vi "Dialog_TestGC (SubVI).vi"() -> ()   [LabVIEW 2017]
uses:
  Global_SNK3_HF.vi
  LV_Unicorn/LV_Unicorn.lvlib
panel:
  in  "Атт":u16(ring) items=["0 дБ"=114, "10 дБ"=104, "20 дБ"=94, "30 дБ"=84, "40 дБ"=74, "50 дБ"=64, "60 дБ"=54, "70 дБ"=44, "80 дБ"=34, "90 дБ"=24, "100 дБ"=14, "110 дБ"=4]
  in  "K":dbl
  in  "K_start":dbl min=0.0 max=80.0
  out "Process":bool
  in  "K_finish":dbl=41.0 format="%#_13g"
  in  "Pause":u32=1000 caption="Пауза, мс"
  out "Meas":bool
  out "subarray 3":sgl[](array[numeric])
  out "subarray 2":sgl[](array[numeric])
  in  "ResetCalCoeff":bool
  in  "index":i32=1 min=1 max=2 step=1
  out "subarray":sgl[](array[numeric])
  in  "WriteCalCoeff":bool
  in  "ReadCalCoeff":bool
  in  "StopMeas":bool
  in  "StartMeas":bool
  in  "Exit":bool
  in  "Coeff":bool
  in  "Tab Control":enum32{"Page 1", "Page 2", "Page 3"}(tab)
  out "TimeMeasStart":u32
  out "Gain0":dbl caption="Усиление 1, дБ" min=0.0 max=80.0 step=1.0 format="%.1g"
  out "Gain1":dbl caption="Усиление 2, дБ" min=0.0 max=80.0 step=1.0 format="%.1g"
  in  "Tick":i32=1 caption="№ такта" min=1 max=32 step=1
  out "TableMeasAmpl":string[][](table)=[["0.000000E+0", "2.352698E-3", "2.352698E-3"], ["1.000000E+0", "2.227753E-3", "2.227753E-3"], ["2.000000E+0", "2.159166E-3", "2.159166E-3"], ["3.000000E+0", "2.145925E-3", "2.145925E-3"], ["4.000000E+0", "2.185622E-3", "2.185622E-3"], ["5.000000E+0", "2.219339E-3", "2.219339E-3"], ["6.000000E+0", "2.237044E-3", "2.237044E-3"], ["7.000000E+0", "2.206156E-3", "2.206156E-3"], ["8.000000E+0", "2.176003E-3", "2.176003E-3"], ["9.000000E+0", "2.179087E-3", "2.179087E-3"], ["1.000000E+1", "2.224777E-3", "2.224777E-3"], ["1.100000E+1", "2.236265E-3", "2.236265E-3"], ["1.200000E+1", "2.240637E-3", "2.240637E-3"], ["1.300000E+1", "2.236521E-3", "2.236521E-3"], ["1.400000E+1", "2.209496E-3", "2.209496E-3"], ["1.500000E+1", "2.200976E-3", "2.200976E-3"], ["1.600000E+1", "2.243053E-3", "2.243053E-3"], ["1.700000E+1", "2.254625E-3", "2.254625E-3"], ["1.800000E+1", "2.279993E-3", "2.279993E-3"], ["1.900000E+1", "2.248004E-3", "2.248004E-3"], ["2.000000E+1", "2.239042E-3", "2.239042E-3"], ["2.100000E+1", "2.234369E-3", "2.234369E-3"], ["2.200000E+1", "2.262064E-3", "2.262064E-3"], ["2.300000E+1", "2.298454E-3", "2.298454E-3"], ["2.400000E+1", "2.297119E-3", "2.297119E-3"], ["2.500000E+1", "2.286266E-3", "2.286266E-3"], ["2.600000E+1", "2.257747E-3", "2.257747E-3"], ["2.700000E+1", "2.267244E-3", "2.267244E-3"], ["2.800000E+1", "2.308694E-3", "2.308694E-3"], ["2.900000E+1", "2.314665E-3", "2.314665E-3"], ["3.000000E+1", "2.329444E-3", "2.329444E-3"], ["3.100000E+1", "2.315041E-3", "2.315041E-3"], ["3.200000E+1", "2.303474E-3", "2.303474E-3"], ["3.300000E+1", "2.340175E-3", "2.340175E-3"], ["3.400000E+1", "2.384913E-3", "2.384913E-3"], ["3.500000E+1", "2.422117E-3", "2.422117E-3"], ["3.600000E+1", "2.405179E-3", "2.405179E-3"], ["3.700000E+1", "2.373606E-3", "2.373606E-3"], ["3.800000E+1", "2.375906E-3", "2.375906E-3"], ["3.900000E+1", "2.410228E-3", "2.410228E-3"], ["4.000000E+1", "2.466864E-3", "2.466864E-3"]]
  in  "GainSlopePL0":sgl=48.8 format="%_4g"
  in  "GainSlopePL1":sgl=48.8 format="%_4g"
  in  "GainOffsetPL0":sgl=1.12 format="%_4g"
  in  "GainOffsetPL1":sgl=1.12 format="%_4g"
  out "Time":u32
  out "Bode":cluster{dbl[], dbl[]}[](graph) caption="XY Graph - Dark"
  out "Array":sgl[][](array[numeric])
  out "GainCorrectionMeas":dbl[][](array[numeric])=[[0.0, 1.0, 2.0, 3.0, 4.0, 5.0, 6.0, 7.0, 8.0, 9.0, 10.0, 11.0, 12.0, 13.0, 14.0, 15.0, 16.0, 17.0, 18.0, 19.0, 20.0, 21.0, 22.0, 23.0, 24.0, 25.0, 26.0, 27.0, 28.0, 29.0, 30.0, 31.0, 32.0, 33.0, 34.0, 35.0, 36.0, 37.0, 38.0, 39.0, 40.0], [-11.232429740269282, -12.70452761402231, -11.319398282381112, -8.995224772277945, -8.870021411520888, -9.034168301334523, -6.792608737521233, -6.370422166599608, -5.823648015304537, -3.66807443072101, -3.031280637510223, -2.0516253300602667, -2.1317894897174536, 0.4940671061840171, 0.61634452640758, 1.0717510423645895, 4.213932160484772, 4.150072217304057, 4.823706052399056, 6.634471019075436, 7.0919550396868996, 8.35048456573561, 10.394659114064568, 10.34651220779031, 10.155847449848958, 11.22080285980282, 12.73098000476622, 13.476154286586526, 13.37702273588783, 15.066209323545356, 16.361307543145575, 17.17482761716563, 17.245659942964423, 18.27256109717559, 18.698807995907593, 18.073313398218705, 18.77836596615101, 19.022884569212057, 18.781051489757388, 19.253641064117456, 20.313889900641513], [-0.02984003478187235, 0.024395588662363472, -0.026881785088726566, -0.01479701311601106, 0.0070473626365402334, -0.04659877911303749, -0.016585774038287197, -0.035195931797667335, 0.018367098970756415, -0.011084536358572277, 0.01184492173421488, 0.008921059976523088, -0.0014462769298614377, -0.010460598191466323, 0.007060342982912368, 0.007319953984052665, 0.0004817943251253796, -0.008217073037779824, 0.010773518388668994, -0.02068839120505336, -0.021134773648135673, 0.007815399845050284, -0.0006033387891328663, -0.009914345630571161, -0.001809363536513138, 0.01397513427572345, 0.011453140739196645, 0.007103610944255908, 0.00231083143198487, -0.0019520005509407457, 0.008239472023896544, 0.011243188031017266, 0.017396690794598844, -0.004540671429712696, 0.003022227667659586, 0.0065086953679980054, 0.05257819699592949, -0.004117202098556384, 0.012485662438209155, 0.02089110110227745, -0.004640054097832816]]
  out "Array 2":sgl[][](array[numeric])
  in  "ClearTableMeasAmpl":bool
  in  "ViewGraf":bool
  in  "ToExcelTable":bool
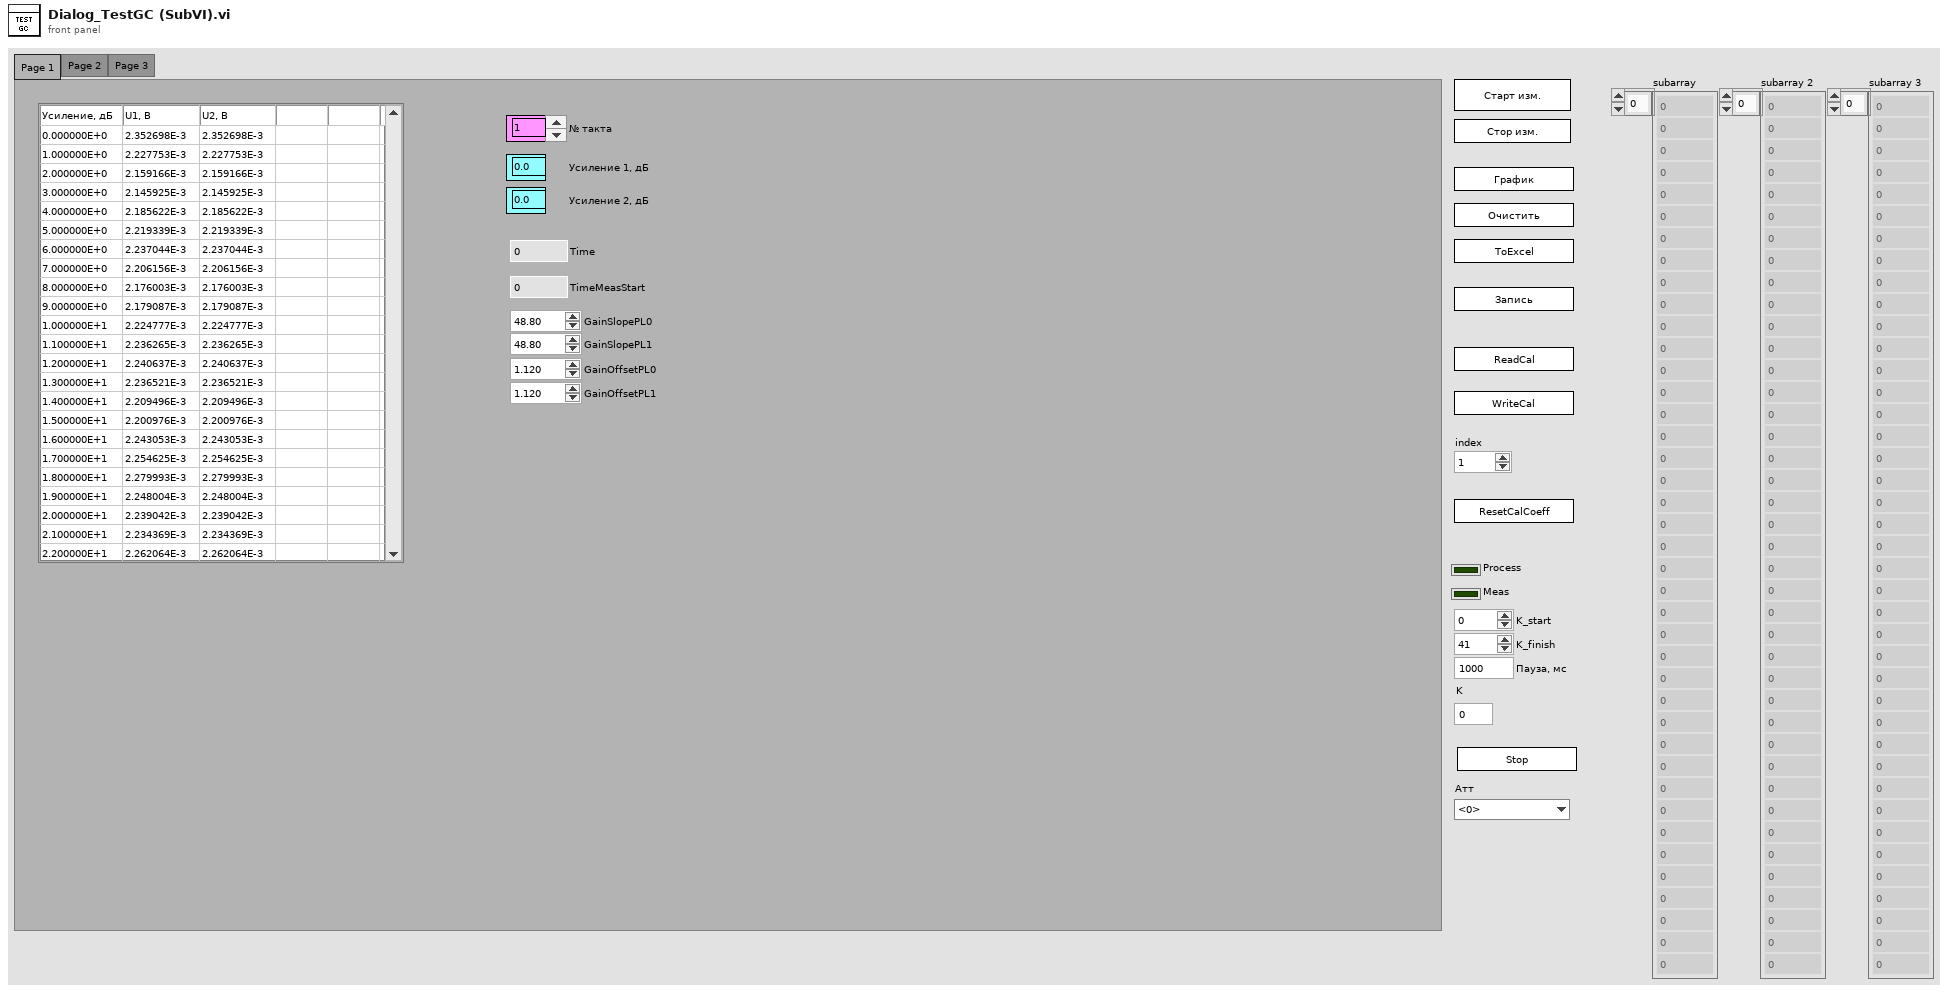
[diagram p1: front panel]
types:
  T1 = typedef "MeasControl.ctl" = cluster{"FFT amplitude":dbl, "amplitude":dbl, "RMS":dbl, "detected frequency":dbl, "way sensor 1":ext, "way sensor 2":ext, "detected frequency 2":dbl, "time trig":dbl, "time trig 2":dbl, "DC":dbl, "trigger detected?":bool, "FFT amplitude mean":dbl}
  T2 = typedef "LV_Unicorn.lvlib/unicorn_Param.ctl" = cluster{"conParam":T3, "Param":T4}
  T3 = typedef "LV_Unicorn.lvlib/unicorn_conn.ctl" = cluster{"ReadIntParam":bool, "ReadDescrParam":bool, "ReadFloatParam":bool, "debug":bool, "ReadJSON":bool, "IP_address":string, "N_attempts":i32, "type_con":enum16{"Serial", "TCP"}, "MB_address":i32, "VISA":refnum<visa-resource-name>, "connection ID":refnum<k5>, "nameDevices":string, "timeout":i32, "port":u16, "type_version":string, "baud_rate":u32, "VersionControl":bool, "TCP_conn":bool, "WindowSize":i32}
  T4 = typedef "LV_Unicorn.lvlib/unicorn_JSON.ctl" = cluster{"NumParam":cluster{"NTelem":i32, "NInt":i32, "NFloat":i32, "NTable":i32}, "ParamInt":T5, "Telemetry":T6, "Table":T7, "ParamFloat":T8}
  T5 = typedef "LV_Unicorn.lvlib/unicorn_ParamInt.ctl" = cluster{"ID":string, "Num":i32, "Name":string, "Type":string, "Enum":string, "Desc":string, "Unit":string, "Access":string, "FormatStr":string, "Min":i32, "Max":i32}[]
  T6 = typedef "LV_Unicorn.lvlib/unicorn_Telemetry.ctl" = cluster{"ID":string, "Num":i32, "Name":string, "Desc":string, "Unit":string, "FormatStr":string, "Min":i32, "Max":i32}[]
  T7 = typedef "LV_Unicorn.lvlib/unicorn_Table.ctl" = cluster{"Num":i32, "Access":string, "ColumnCount":i32, "NeedParamPrepare":bool, "Columns":cluster{"Column":i32, "Desc":string, "Name":string}[], "DataType":string, "FormatStr":string, "ID":string, "Name":string, "RowCount":i32, "Rows":cluster{"Desc":string, "ID":string, "Max":i32, "Min":i32, "Name":string, "Row":i32, "Unit":string}[], "Type":string}[]
  T8 = typedef "LV_Unicorn.lvlib/unicorn_ParamFloat.ctl" = cluster{"ID":string, "Num":i32, "Name":string, "Type":string, "Enum":string, "Desc":string, "Unit":string, "Access":string, "FormatStr":string, "Min":sgl, "Max":sgl}[]
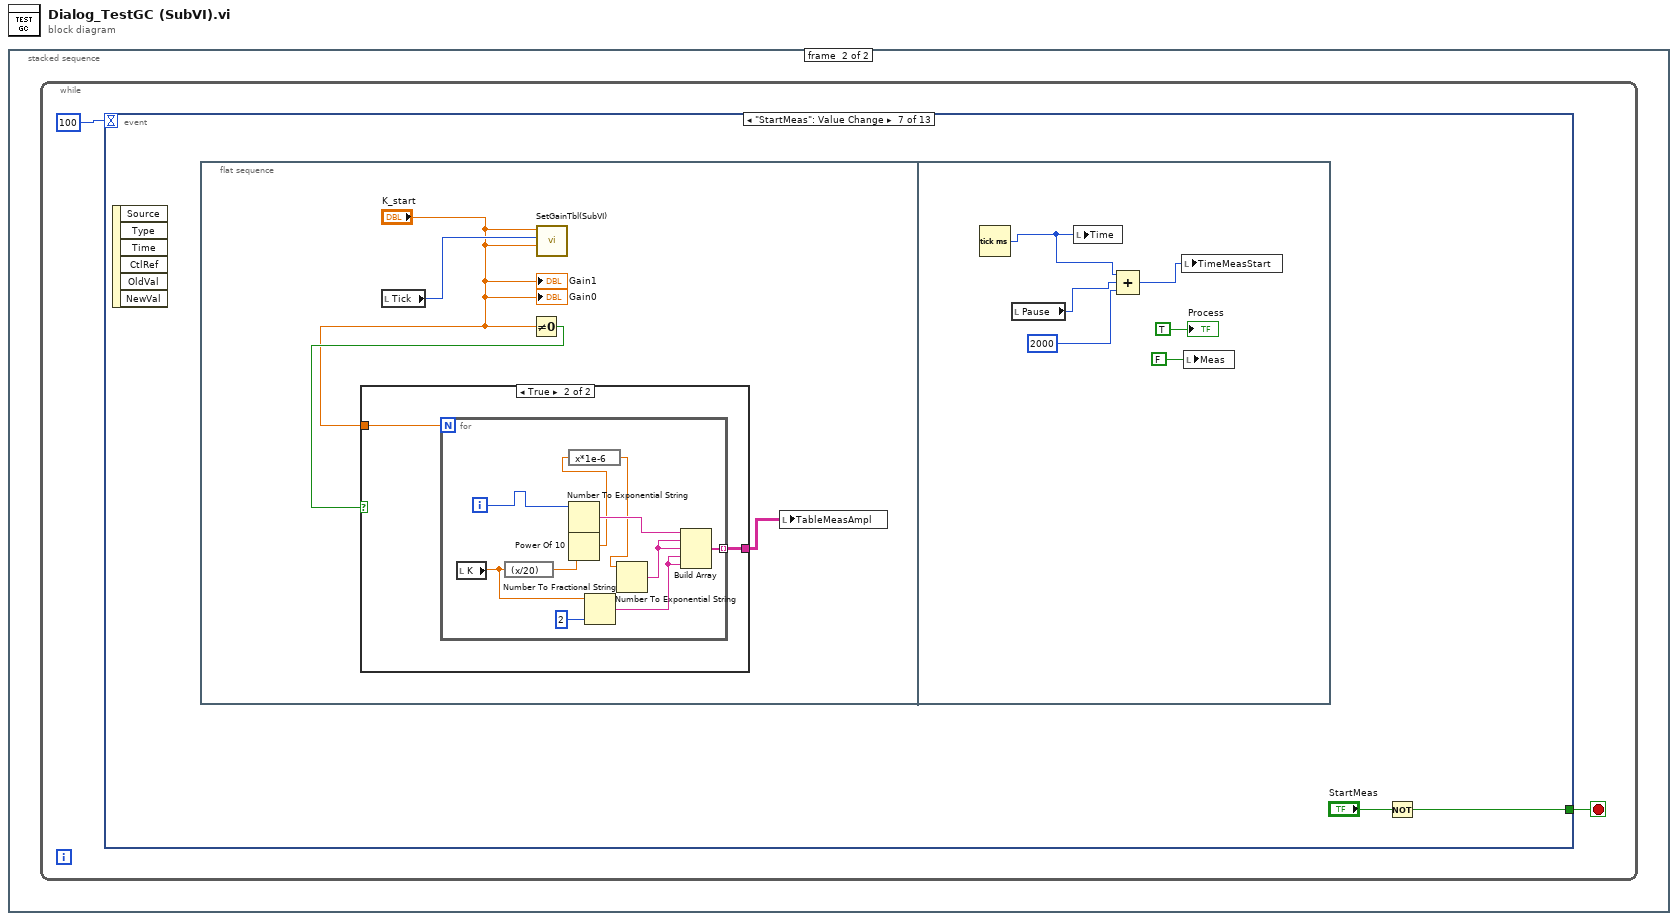
[diagram p0: block diagram]
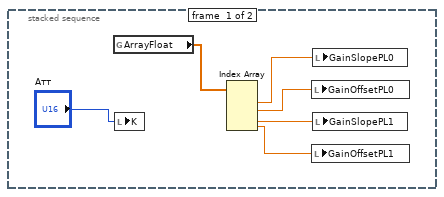
[diagram p2: hidden frame]
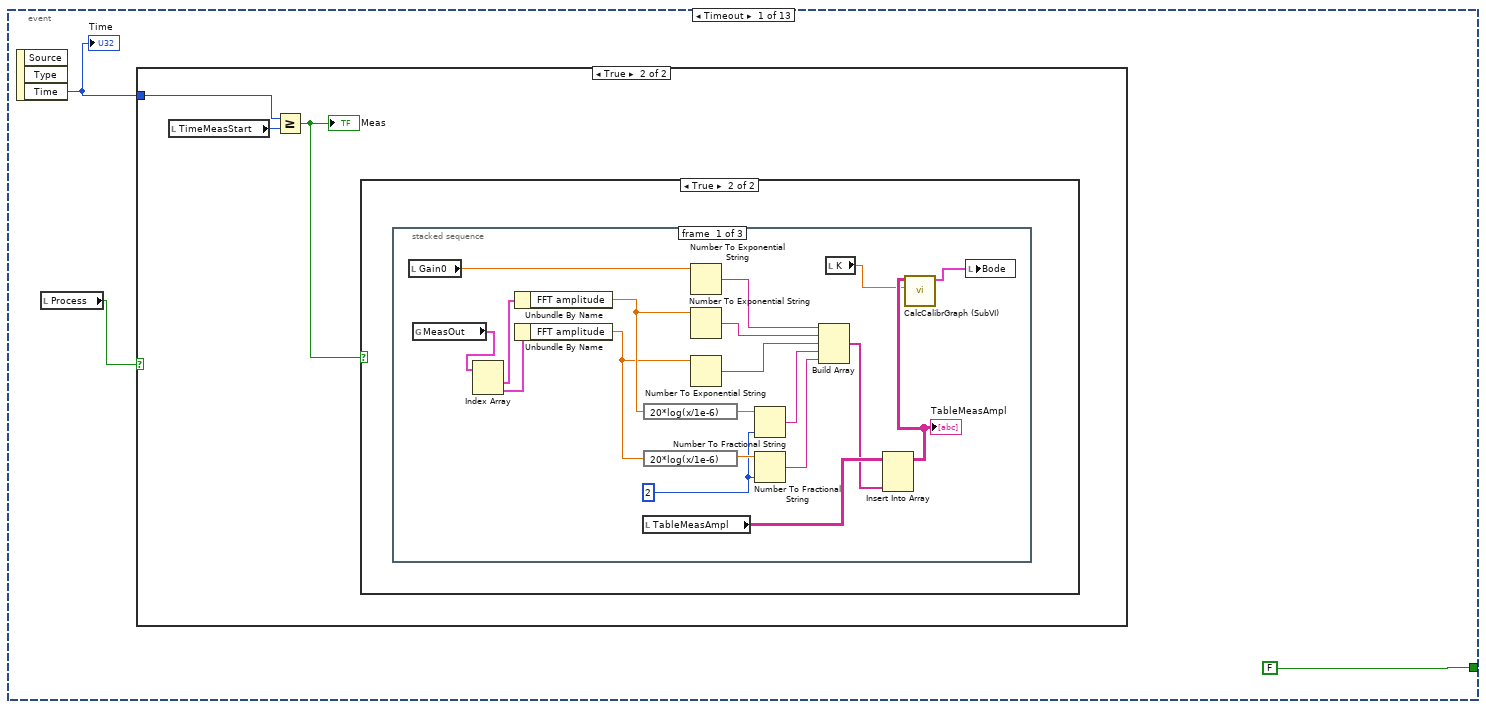
[diagram p3: hidden frame]
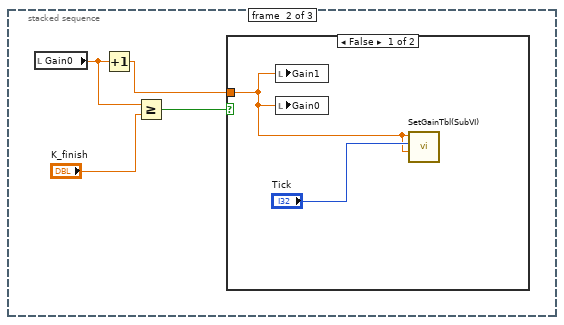
[diagram p6: hidden frame]
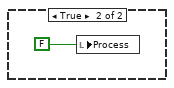
[diagram p7: hidden frame]
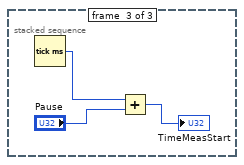
[diagram p8: hidden frame]
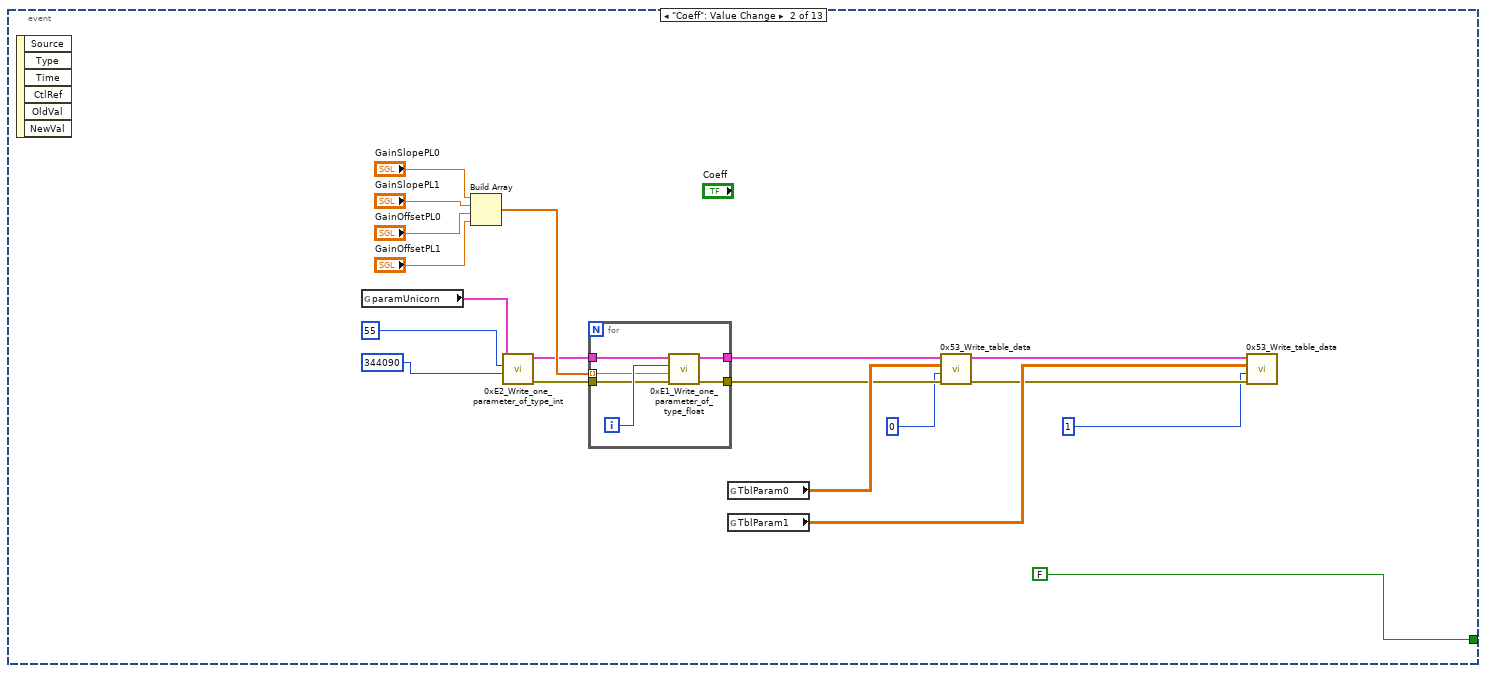
[diagram p9: hidden frame]
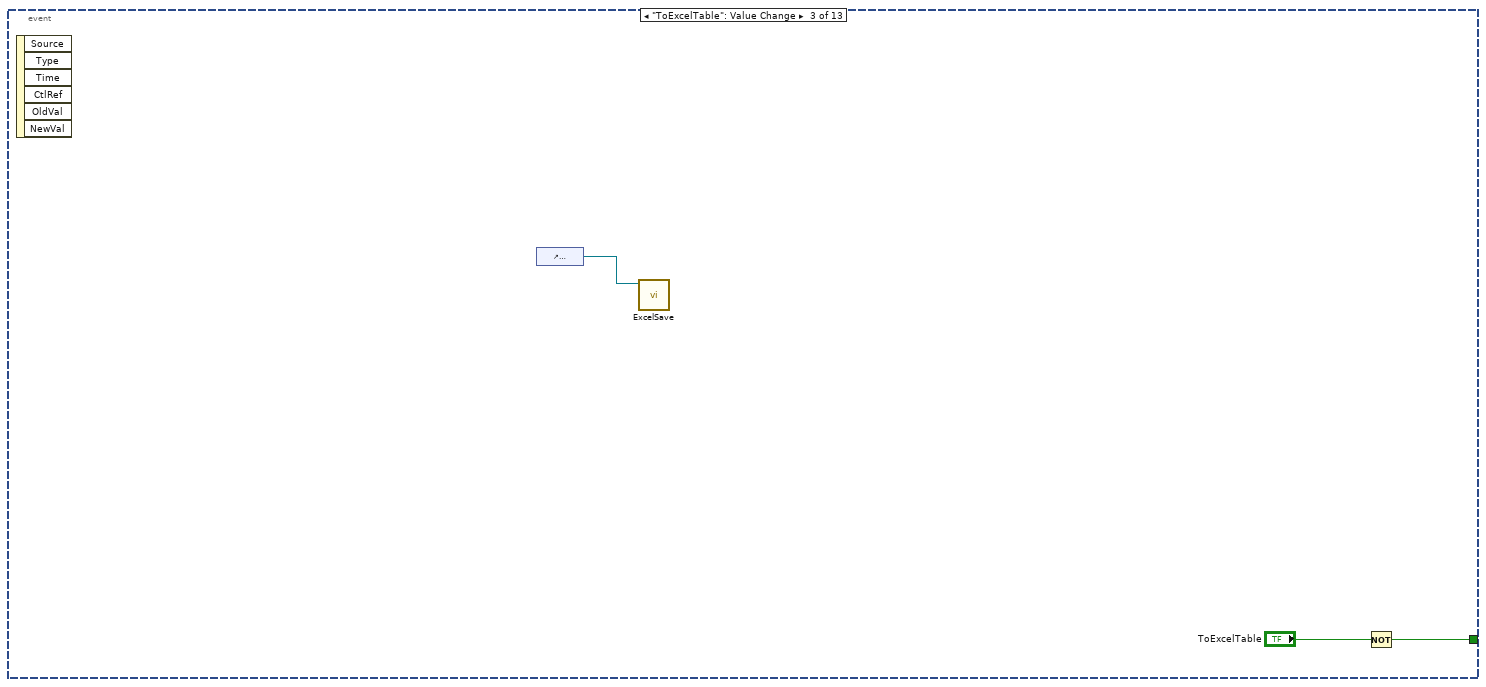
[diagram p10: hidden frame]
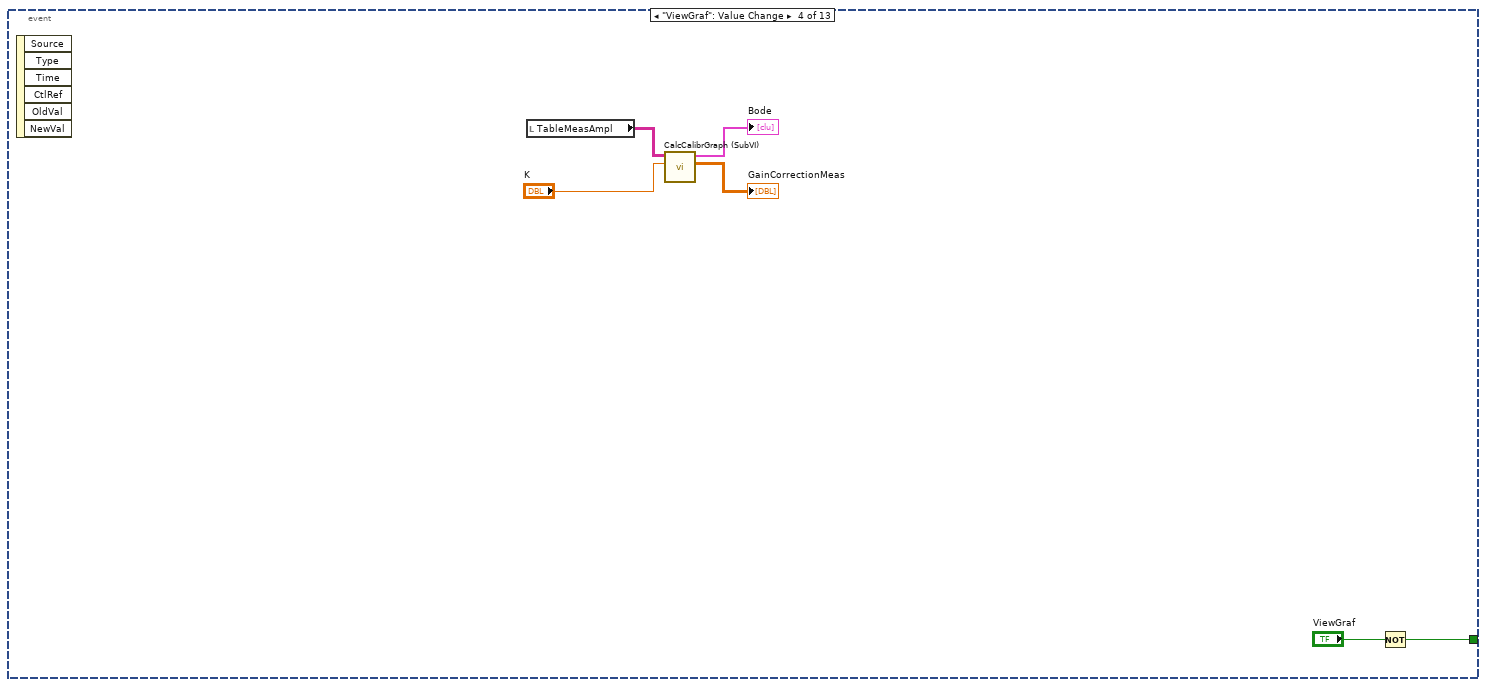
[diagram p11: hidden frame]
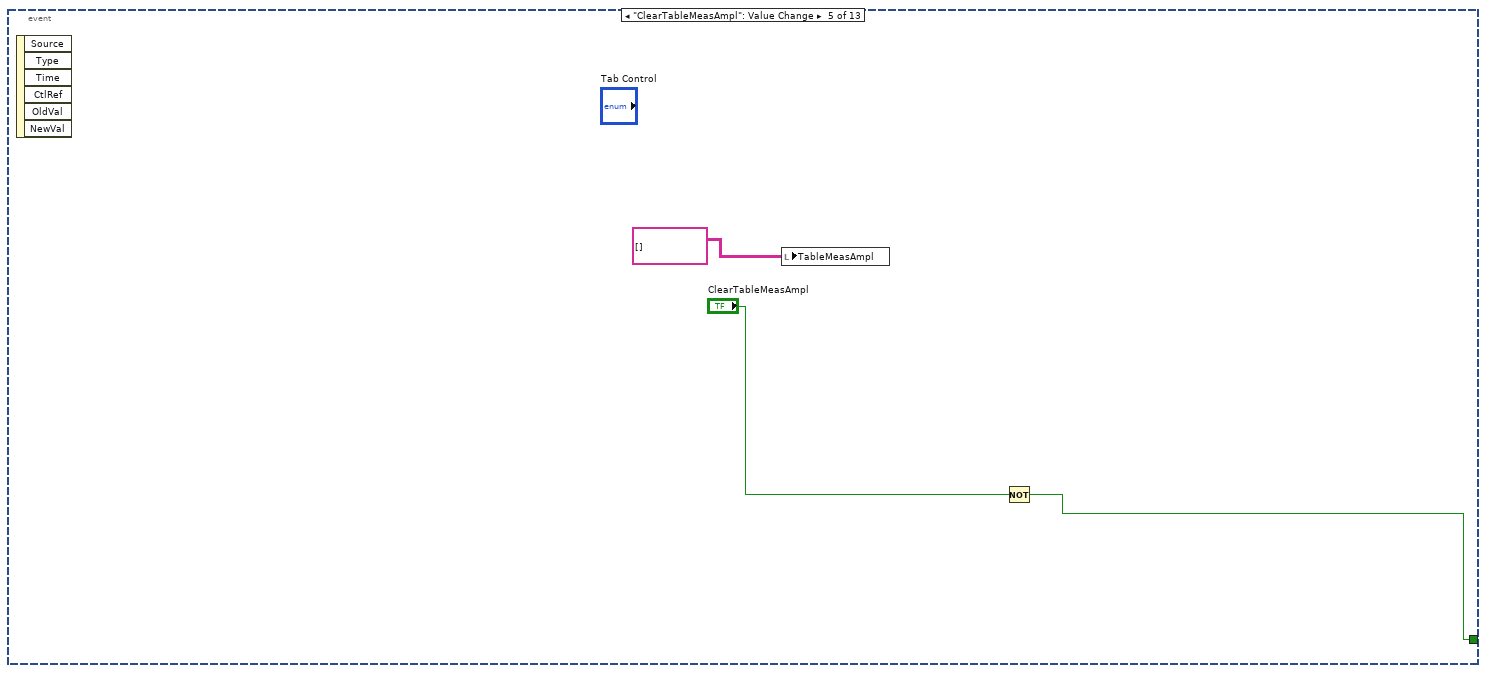
[diagram p12: hidden frame]
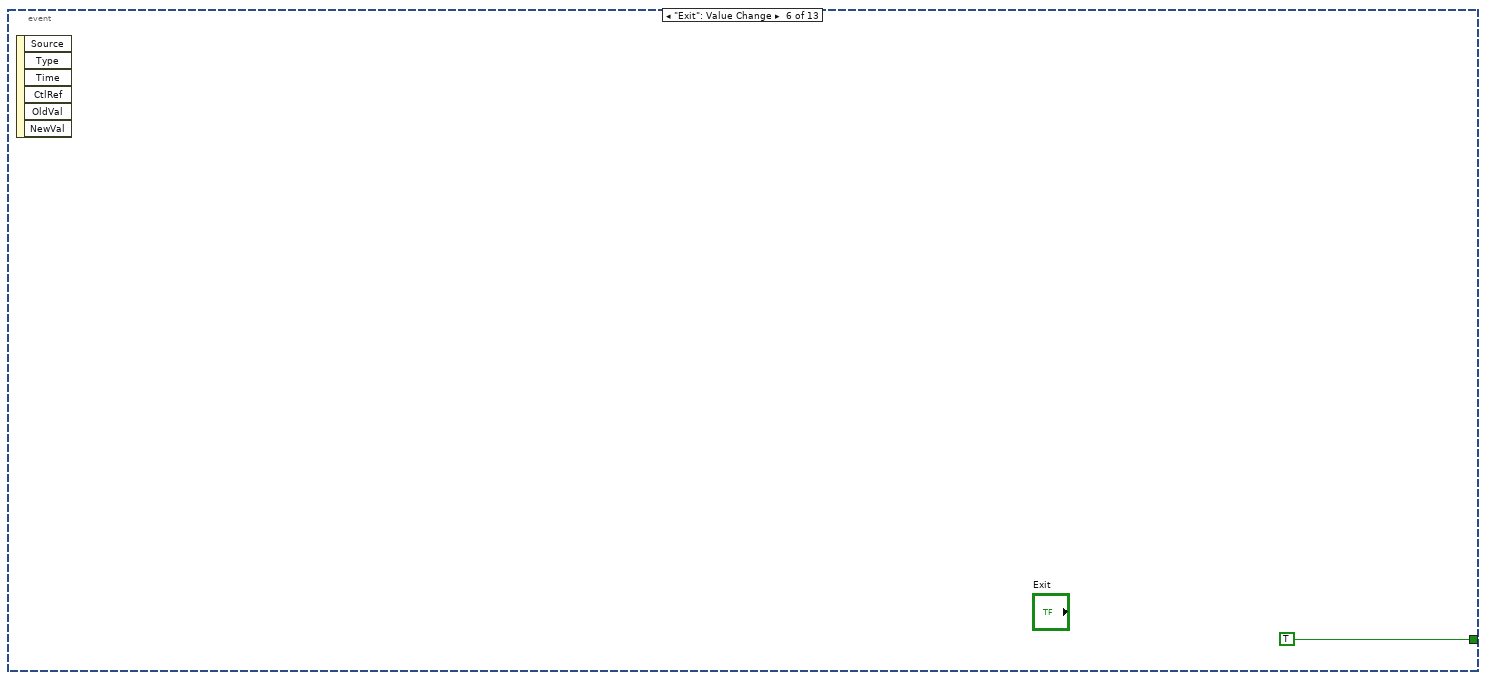
[diagram p13: hidden frame]
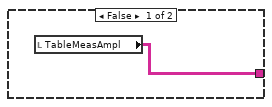
[diagram p14: hidden frame]
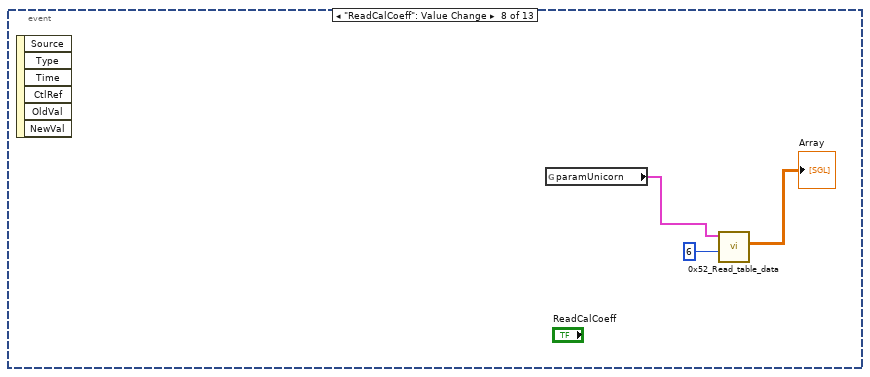
[diagram p15: hidden frame]
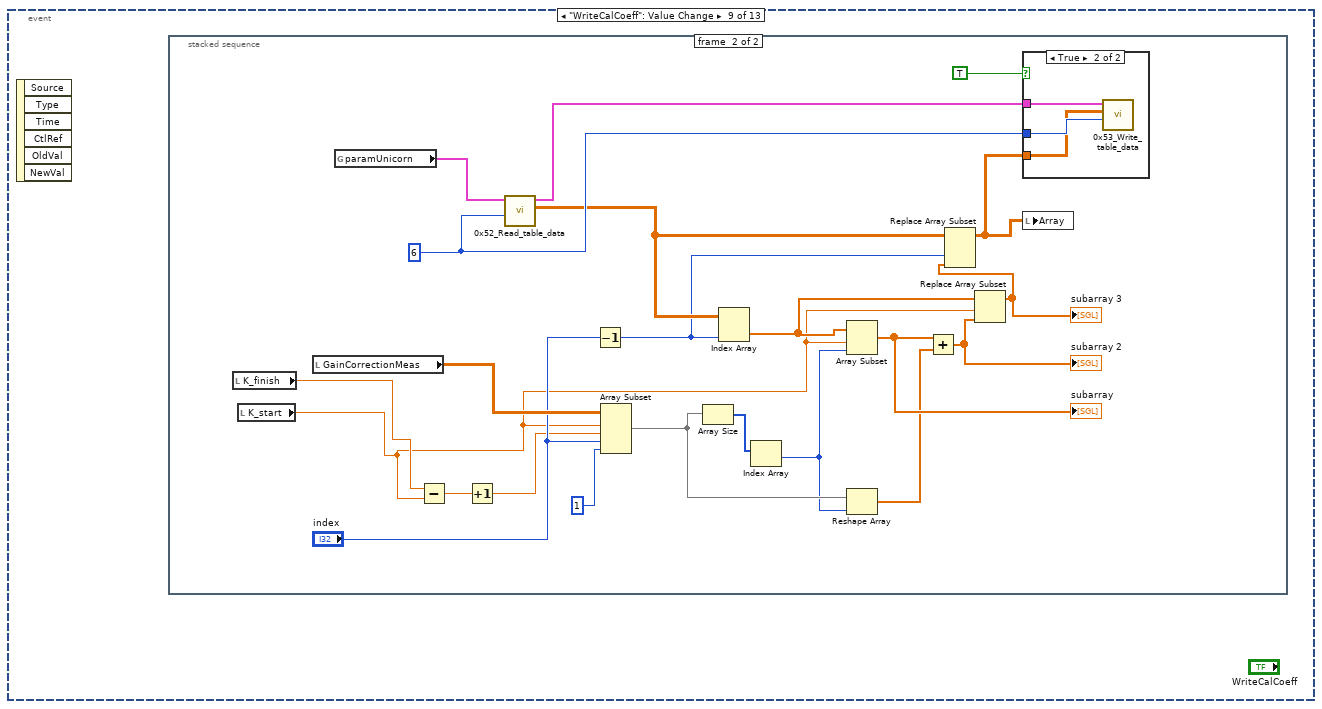
[diagram p16: hidden frame]
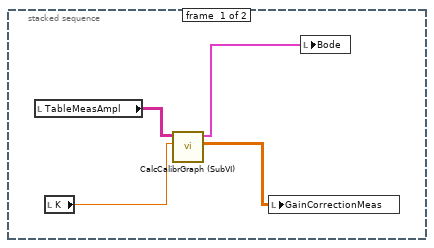
[diagram p17: hidden frame]
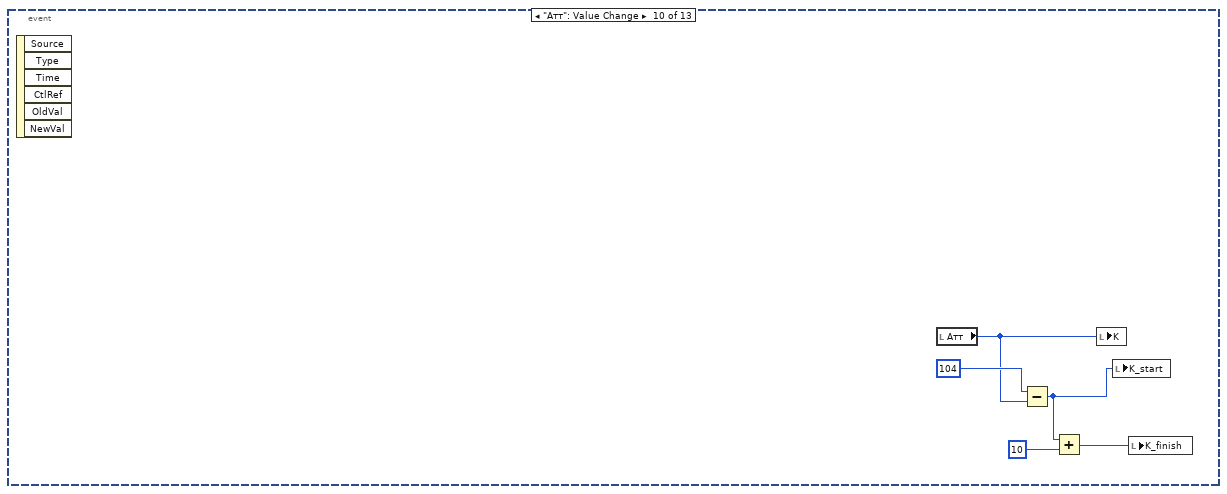
[diagram p19: hidden frame]
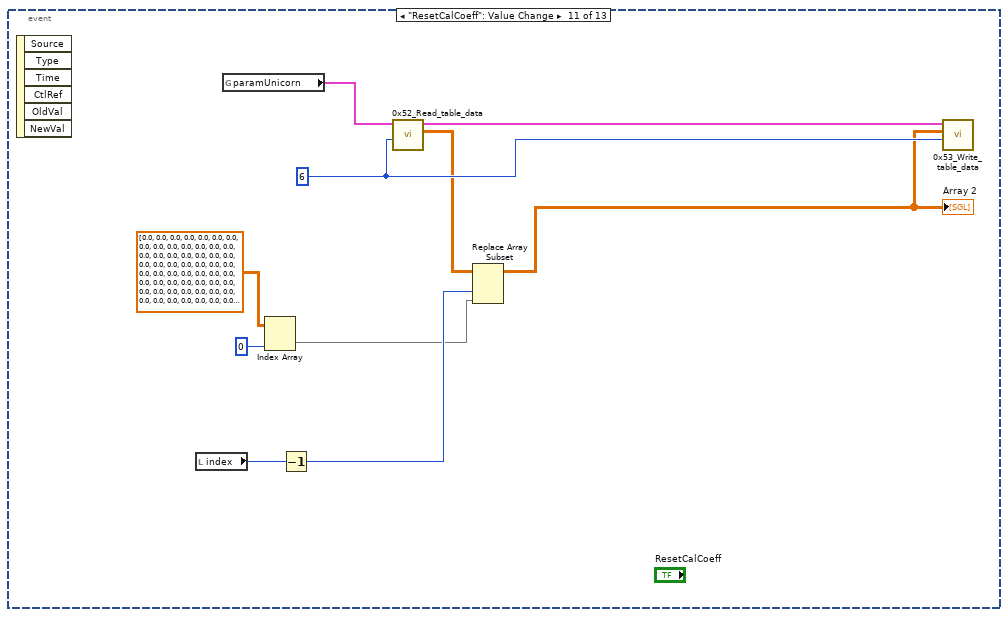
[diagram p20: hidden frame]
diagram:
  n1 = stacked-sequence {
    frame #0 {
      n2 = global read "Global_SNK3_HF.vi" "ArrayFloat"() -> (w2:sgl[])
      n3 = local write "K"("Атт") -> ()
      n4 = Index Array(array=w2) -> (element #1=w6:sgl, element #2=w5:sgl, element #3=w4:sgl, element #4=w3:sgl)  [unwired: 4 in]
      n5 = local write "GainOffsetPL0"(w5) -> ()
      n6 = local write "GainOffsetPL1"(w3) -> ()
      n7 = local write "GainSlopePL0"(w6) -> ()
      n8 = local write "GainSlopePL1"(w4) -> ()
    }
    frame #1 {
      n9 = while {
        stop <- w7 stop-if-true
        n10 = event shown="[6] \"StartMeas\": Value Change" {
          selector: _ -> [_ _ _ _ _ _ _ _ _ _ _ _ _]
          dyn-events: _ -> [_ _ _ _ _ _ _ _ _ _ _ _ _]
          timeout: 100 -> [_ _ _ _ _ _ _ _ _ _ _ _ _]
          tunnel: [FALSE FALSE w69 w74 w78 TRUE w82 _ _ _ _ w156 TRUE] -> w7
          event Timeout {
            n11 = event-data() -> ("Time"=w9:u32)  [unwired: 1 in, 2 out]
            "Time" <- w9
            n12 = local read "Process"() -> (w10:bool)
            n13 = case shown="True" w10 {
              tunnel: w9 -> [_ w13]
              frame False {
              }
              frame True {
                n14 = local read "TimeMeasStart"() -> (w14:u32)
                n15 = Greater Or Equal?(x=w13, y=w14) -> (x >= y?=w12:bool)
                "Meas" <- w12
                n16 = case shown="True" w12 {
                  frame False {
                  }
                  frame True {
                    n17 = stacked-sequence {
                      frame #0 {
                        w21 = i16 2 ("precision (6)")
                        n18 = local read "Gain0"() -> (w32:dbl)
                        n19 = global read "Global_SNK3_HF.vi" "MeasOut"() -> (w20:T1[])
                        n20 = Index Array(array=w20) -> (element #1=w19:T1, element #2=w18:T1)  [unwired: 2 in]
                        n21 = Unbundle By Name(w19) -> ("FFT amplitude"=w27:dbl)
                        n22 = Unbundle By Name(w18) -> ("FFT amplitude"=w26:dbl)
                        n23 = local read "TableMeasAmpl"() -> (w33:string[][])
                        n24 = expression code="20*log(x/1e-6)"(w27) -> (w25:dbl)
                        n25 = expression code="20*log(x/1e-6)"(w26) -> (w24:dbl)
                        n26 = Number To Exponential String(number=w32) -> (E-format string=w31:string)  [unwired: 3 in]
                        n27 = Number To Exponential String(number=w27) -> (E-format string=w30:string)  [unwired: 3 in]
                        n28 = Number To Exponential String(number=w26) -> (E-format string=w29:string)  [unwired: 3 in]
                        n29 = Number To Fractional String(number=w25, precision (6)=w21) -> (F-format string=w23:string)  [unwired: 2 in]
                        n30 = Number To Fractional String(number=w24, precision (6)=w21) -> (F-format string=w22:string)  [unwired: 2 in]
                        n31 = Build Array(w31, w30, w29, w23, w22) -> (w28:string[])
                        n32 = local read "K"() -> (w15:dbl)
                        n33 = Insert Into Array(array=w33, new element=w28) -> (w17:string[][])  [unwired: 2 in]
                        "TableMeasAmpl" <- w17
                        n34 = call "CalcCalibrGraph (SubVI).vi"("K"=w15, "TableMeasAmpl"=w17) -> ("Array"=w16:cluster{dbl[], dbl[]}[])  [unwired: 8 in, 1 out]
                        n35 = local write "Bode"(w16) -> ()
                      }
                      frame #1 {
                        n36 = local read "Gain0"() -> (w35:dbl)
                        n37 = Increment(x=w35) -> (x+1=w37:dbl)
                        n38 = Greater Or Equal?(x=w35, y="K_finish") -> (x >= y?=w34:bool)
                        n39 = case shown="False" w34 {
                          tunnel: w37 -> [w38 _]
                          frame False {
                            n40 = local write "Gain1"(w38) -> ()
                            n41 = local write "Gain0"(w38) -> ()
                            n42 = call "SetGainTbl(SubVI).vi"("Gain0"=w38, "Tick"="Tick", "Gain1"=w38) -> ()  [unwired: 8 in, 1 out]
                          }
                          frame True {
                            n43 = local write "Process"(FALSE ("GainMeas")) -> ()
                          }
                        }
                      }
                      frame #2 {
                        n44 = Tick Count (ms)() -> (millisecond timer value=w41:u32)
                        n45 = Add(x=w41, y="Pause") -> (x+y=→"TimeMeasStart":u32)
                      }
                    }
                  }
                }
              }
            }
          }
          event "Coeff": Value Change {
            n46 = event-data() -> ()  [unwired: 1 in, 6 out]
            n47 = global read "Global_SNK3_HF.vi" "paramUnicorn"() -> (w45:T2)
            n48 = Build Array("GainSlopePL0", "GainSlopePL1", "GainOffsetPL0", "GainOffsetPL1") -> (w55:sgl[])
            n49 = call "0xE2_Write_one_parameter_of_type_int.vi"("ParamIn"=344090 ("Значение параметра"), "NumParamIn"=55 ("Номер параметра"), "paramUnicorn 2"=w45) -> ("error out"=w56:errorcluster, "paramUnicornOut"=w50:T2)  [unwired: 5 in, 2 out]
            n50 = for {
              tunnel: w50 -> [w68]
              tunnel: w55 -> [w66] mode=indexing
              tunnel: w56 -> [w65]
              tunnel: [w64] -> w58
              tunnel: [w63] -> w57
              i -> [w67]
              n51 = call "0xE1_Write_one_parameter_of_type_float.vi"("error in"=w65, "Значение параметра"=w66, "Номер параметра"=w67, "ParamIn"=w68) -> ("error out"=w63:errorcluster, "ParamOut"=w64:T2)  [unwired: 4 in, 2 out]
            }
            n52 = global read "Global_SNK3_HF.vi" "TblParam0"() -> (w61:sgl[][])
            n53 = global read "Global_SNK3_HF.vi" "TblParam1"() -> (w62:sgl[][])
            n54 = call "0x53_Write_table_data.vi"("error in"=w57, "Номер табличного параметра 2"=0, "ArrayIn"=w61, "paramUnicorn"=w58) -> ("error out"=w60:errorcluster, "paramUnicorn 2"=w59:T2)  [unwired: 4 in, 2 out]
            n55 = call "0x53_Write_table_data.vi"("error in"=w60, "Номер табличного параметра 2"=1, "ArrayIn"=w62, "paramUnicorn"=w59) -> ()  [unwired: 4 in, 4 out]
          }
          event "ToExcelTable": Value Change {
            n56 = event-data() -> ()  [unwired: 1 in, 6 out]
            n57 = control-ref of="TableMeasAmpl"() -> (w71:refnum<vi>)
            n58 = call "ExcelSave.vi"("Table in"=w71) -> ()  [unwired: 10 in, 1 out]
            n59 = Not(x="ToExcelTable") -> (.not. x?=w69:bool)
          }
          event "ViewGraf": Value Change {
            n60 = event-data() -> ()  [unwired: 1 in, 6 out]
            n61 = local read "TableMeasAmpl"() -> (w76:string[][])
            n62 = call "CalcCalibrGraph (SubVI).vi"("K"="K", "TableMeasAmpl"=w76) -> ("Array 2"=→"GainCorrectionMeas":dbl[][], "Array"=→"Bode":cluster{dbl[], dbl[]}[])  [unwired: 8 in]
            n63 = Not(x="ViewGraf") -> (.not. x?=w74:bool)
          }
          event "ClearTableMeasAmpl": Value Change {
            n64 = event-data() -> ()  [unwired: 1 in, 6 out]
            n65 = local write "TableMeasAmpl"(string[][] [] ("Таблица телеметрии")) -> ()
            n66 = Not(x="ClearTableMeasAmpl") -> (.not. x?=w78:bool)
          }
          event "Exit": Value Change {
            n67 = event-data() -> ()  [unwired: 1 in, 6 out]
          }
          event "StartMeas": Value Change {
            n68 = event-data() -> ()  [unwired: 1 in, 6 out]
            n69 = flat-sequence {
              frame #0 {
                n70 = local read "Tick"() -> (w87:i32)
                n71 = Not Equal To 0?(x="K_start") -> (x != 0?=w86:bool)
                n72 = case shown="True" w86 {
                  tunnel: "K_start" -> [_ w89]
                  tunnel: [w88 w90] -> w84
                  frame False {
                    n73 = local read "TableMeasAmpl"() -> (w88:string[][])
                  }
                  frame True {
                    n74 = for {
                      N: w89 -> [_]
                      tunnel: [w95] -> w90 mode=indexing
                      i -> [w91]
                      n75 = local read "K"() -> (w98:dbl)
                      n76 = expression code="(x/20)"(w98) -> (w94:dbl)
                      n77 = Number To Exponential String(number=w91) -> (E-format string=w100:string)  [unwired: 3 in]
                      n78 = Power Of 10(x=w94) -> (10^x=w93:dbl)
                      n79 = expression code="x*1e-6"(w93) -> (w92:dbl)
                      n80 = Number To Fractional String(number=w98, precision (6)=i16 2) -> (F-format string=w96:string)  [unwired: 2 in]
                      n81 = Number To Exponential String(number=w92) -> (E-format string=w99:string)  [unwired: 3 in]
                      n82 = Build Array(w100, w99, w99, w96, w96) -> (w95:string[])
                    }
                  }
                }
                n83 = call "SetGainTbl(SubVI).vi"("Gain0"="K_start", "Tick"=w87, "Gain1"="K_start") -> ()  [unwired: 8 in, 1 out]
                n84 = local write "TableMeasAmpl"(w84) -> ()
                "Gain0" <- "K_start"
                "Gain1" <- "K_start"
              }
              frame #1 {
                n85 = Tick Count (ms)() -> (millisecond timer value=w104:u32)
                n86 = local read "Pause"() -> (w106:u32)
                n87 = local write "Time"(w104) -> ()
                n88 = Compound Arithmetic op=ADD(w104, w106, u32 2000 ("value")) -> (w105:u32)
                n89 = local write "TimeMeasStart"(w105) -> ()
                n90 = local write "Meas"(FALSE ("Meas")) -> ()
                "Process" <- TRUE ("Process")
              }
            }
            n91 = Not(x="StartMeas") -> (.not. x?=w82:bool)
          }
          event "ReadCalCoeff": Value Change {
            n92 = event-data() -> ()  [unwired: 1 in, 6 out]
            n93 = global read "Global_SNK3_HF.vi" "paramUnicorn"() -> (w109:T2)
            n94 = call "0x52_Read_table_data.vi"("NTable"=6, "paramUnicornIn"=w109) -> ("Array"=→"Array":sgl[][])  [unwired: 7 in, 2 out]
          }
          event "WriteCalCoeff": Value Change {
            n95 = event-data() -> ()  [unwired: 1 in, 6 out]
            n96 = stacked-sequence {
              frame #0 {
                n97 = local read "TableMeasAmpl"() -> (w110:string[][])
                n98 = local read "K"() -> (w113:dbl)
                n99 = call "CalcCalibrGraph (SubVI).vi"("K"=w113, "TableMeasAmpl"=w110) -> ("Array 2"=w111:dbl[][], "Array"=w112:cluster{dbl[], dbl[]}[])  [unwired: 8 in]
                n100 = local write "GainCorrectionMeas"(w111) -> ()
                n101 = local write "Bode"(w112) -> ()
              }
              frame #1 {
                w134 = 6 ("NTable")
                n102 = local read "K_finish"() -> (w115:dbl)
                n103 = local read "K_start"() -> (w114:dbl)
                n104 = local read "GainCorrectionMeas"() -> (w132:dbl[][])
                n105 = global read "Global_SNK3_HF.vi" "paramUnicorn"() -> (w135:T2)
                n106 = Subtract(x=w115, y=w114) -> (x-y=w117:dbl)
                n107 = Increment(x=w117) -> (x+1=w116:dbl)
                n108 = call "0x52_Read_table_data.vi"("NTable"=w134, "paramUnicornIn"=w135) -> ("Array"=w127:sgl[][], "paramUnicornOut"=w133:T2)  [unwired: 7 in, 1 out]
                n109 = Decrement(x="index") -> (x-1=w126:i32)
                n110 = Array Subset(array=w132, index (row)=w114, length (row)=w116, index (col)="index", length (col)=1 ("index")) -> (w130:dbl[][])
                n111 = Array Size(array=w130) -> (size(s)=w129:i32[])
                n112 = Index Array(array=w127, index (col)=w126) -> (element=w122:sgl[])  [unwired: 1 in]
                n113 = Index Array(array=w129) -> (element=w124:i32)  [unwired: 1 in]
                n114 = Array Subset(array=w122, index=w114, length=w124) -> (w121:sgl[])
                "subarray" <- w121
                n115 = Reshape Array(w130, w124) -> (w120:dbl[])
                n116 = Add(x=w121, y=w120) -> (x+y=w119:dbl[])
                "subarray 2" <- w119
                n117 = Replace Array Subset(array=w122, new element=w119, index=w114) -> (w118:sgl[])
                "subarray 3" <- w118
                n118 = Replace Array Subset(array=w127, new element=w118, index (col)=w126) -> (w125:sgl[][])  [unwired: 1 in]
                n119 = case shown="True" TRUE {
                  tunnel: w134 -> [_ w138]
                  tunnel: w133 -> [_ w137]
                  tunnel: w125 -> [_ w136]
                  frame False {
                  }
                  frame True {
                    n120 = call "0x53_Write_table_data.vi"("Номер табличного параметра 2"=w138, "ArrayIn"=w136, "paramUnicorn"=w137) -> ()  [unwired: 5 in, 4 out]
                  }
                }
                n121 = local write "Array"(w125) -> ()
              }
            }
          }
          event "Атт": Value Change {
            n122 = event-data() -> ()  [unwired: 1 in, 6 out]
            n123 = local read "Атт"() -> (w142:u16)
            n124 = Subtract(x=104, y=w142) -> (x-y=w140:i32)
            n125 = Add(x=w140, y=10) -> (x+y=w139:i32)
            n126 = local write "K"(w142) -> ()
            n127 = local write "K_start"(w140) -> ()
            n128 = local write "K_finish"(w139) -> ()
          }
          event "ResetCalCoeff": Value Change {
            w151 = 6 ("NTable")
            n129 = event-data() -> ()  [unwired: 1 in, 6 out]
            n130 = local read "index"() -> (w150:i32)
            n131 = global read "Global_SNK3_HF.vi" "paramUnicorn"() -> (w153:T2)
            n132 = Index Array(array=sgl[][] [[0.0, 0.0], [0.0, 0.0], [0.0, 0.0], [0.0, 0.0], [0.0, 0.0], [0.0, 0.0], [0.0, 0.0], [0.0, 0.0], [0.0, 0.0], [0.0, 0.0], [0.0, 0.0], [0.0, 0.0], [0.0, 0.0], [0.0, 0.0], [0.0, 0.0], [0.0, 0.0], [0.0, 0.0], [0.0, 0.0], [0.0, 0.0], [0.0, 0.0], [0.0, 0.0], [0.0, 0.0], [0.0, 0.0], [0.0, 0.0], [0.0, 0.0], [0.0, 0.0], [0.0, 0.0], [0.0, 0.0], [0.0, 0.0], [0.0, 0.0], [0.0, 0.0], [0.0, 0.0], [0.0, 0.0], [0.0, 0.0], [0.0, 0.0], [0.0, 0.0], [0.0, 0.0], [0.0, 0.0], [0.0, 0.0], [0.0, 0.0], [0.0, 0.0], [0.0, 0.0], [0.0, 0.0], [0.0, 0.0], [0.0, 0.0], [0.0, 0.0], [0.0, 0.0], [0.0, 0.0], [0.0, 0.0], [0.0, 0.0], [0.0, 0.0], [0.0, 0.0], [0.0, 0.0], [0.0, 0.0], [0.0, 0.0], [0.0, 0.0], [0.0, 0.0], [0.0, 0.0], [0.0, 0.0], [0.0, 0.0], [0.0, 0.0], [0.0, 0.0], [0.0, 0.0], [0.0, 0.0], [0.0, 0.0], [0.0, 0.0], [0.0, 0.0], [0.0, 0.0], [0.0, 0.0], [0.0, 0.0], [0.0, 0.0], [0.0, 0.0], [0.0, 0.0], [0.0, 0.0], [0.0, 0.0], [0.0, 0.0], [0.0, 0.0], [0.0, 0.0], [0.0, 0.0], [0.0, 0.0], [0.0, 0.0]] ("Array 2"), index (col)=0 ("disabled index (col)")) -> (element=w145:sgl[])  [unwired: 1 in]
            n133 = Decrement(x=w150) -> (x-1=w146:i32)
            n134 = call "0x52_Read_table_data.vi"("NTable"=w151, "paramUnicornIn"=w153) -> ("Array"=w147:sgl[][], "paramUnicornOut"=w152:T2)  [unwired: 7 in, 1 out]
            n135 = Replace Array Subset(array=w147, new element=w145, index (col)=w146) -> (w144:sgl[][])  [unwired: 1 in]
            "Array 2" <- w144
            n136 = call "0x53_Write_table_data.vi"("Номер табличного параметра 2"=w151, "ArrayIn"=w144, "paramUnicorn"=w152) -> ()  [unwired: 5 in, 4 out]
          }
          event "StopMeas": Value Change {
            n137 = event-data() -> ()  [unwired: 1 in, 6 out]
            n138 = local write "Process"(FALSE ("Process")) -> ()
            n139 = local write "Meas"(FALSE ("GainMeas")) -> ()
            n140 = Not(x="StopMeas") -> (.not. x?=w156:bool)
          }
          event Panel Close? {
            n141 = event-data() -> ()  [unwired: 1 in, 4 out]
            n142 = event-data() -> ()  [unwired: 2 in, 1 out]
          }
        }
      }
    }
  }
